vi "Sort Inductance Matrix.vi"(1 "Current sorted?":cluster{"Id sorted?":bool, "Iq sorted?":bool}, 3 "Inductance Matrix in":dbl[][](array[numeric])) -> (0 "Inductance Matrix out":dbl[][](array[numeric]))   [LabVIEW 2019]
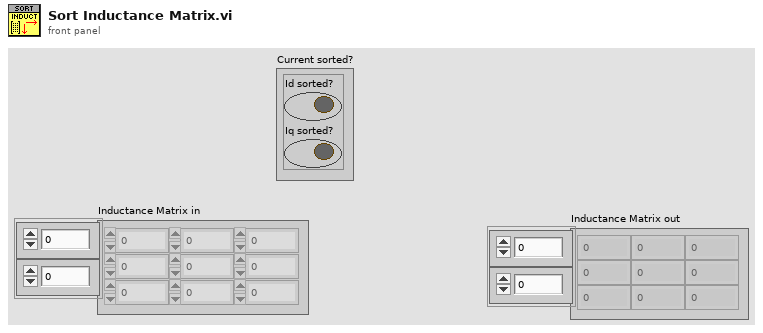
[diagram p1: front panel]
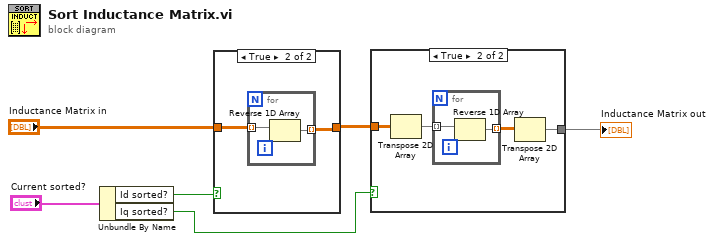
[diagram p0: block diagram]
diagram:
  n1 = Unbundle By Name("Current sorted?") -> ("Id sorted?"=w4:bool, "Iq sorted?"=w2:bool)
  n2 = case shown="True" w4 {
    tunnel: "Inductance Matrix in" -> [w7 w9]
    tunnel: [w7 w8] -> w3
    frame False {
    }
    frame True {
      n3 = for {
        tunnel: w9 -> [w11] mode=indexing
        tunnel: [w10] -> w8 mode=indexing
        n4 = Reverse 1D Array(array=w11) -> (reversed array=w10:dbl[])
      }
    }
  }
  n5 = case shown="True" w2 {
    tunnel: w3 -> [w12 w14]
    tunnel: [w12 w15] -> w1
    frame False {
    }
    frame True {
      n6 = Transpose 2D Array(2D array=w14) -> (transposed array=w13:dbl[][])
      n7 = for {
        tunnel: w13 -> [w18] mode=indexing
        tunnel: [w17] -> w16 mode=indexing
        n8 = Reverse 1D Array(array=w18) -> (reversed array=w17:dbl[])
      }
      n9 = Transpose 2D Array(2D array=w16) -> (transposed array=w15:dbl[][])
    }
  }
  "Inductance Matrix out" <- w1
